vi "EZ1 MB1010 Sonar - Digital.vi"() -> ()   [LabVIEW 2013]
doc: "This example shows how to use the MaxBotix LV-MaxSonar-EZ1 Sonar Range Finder MB1010. It will display the distance from the sensor in inches.\n\nThis example works with the NI 9403 module connected to a Digital Sidecar. The Digital Sidecar should have 12V applied to the WAGO connector. The sensor is attached to the 3x8 header using a 3-pin PWM connector."
uses:
  <vilib>/Rock Robotics/SystemInterfaces/DIO/FPGA_DIOChannel.ctl
  <vilib>/Rock Robotics/SystemInterfaces/Typedef/FPGA_TypedefDigitalModule.ctl
  <vilib>/Rock Robotics/WPI/Counter/WPI_CounterDigitalInputToDigitalSource.vi
  <vilib>/Rock Robotics/WPI/Counter/WPI_CounterOpen Semi Period Mode.vi
panel:
  out "distance":dbl(slide)=125.0 scale=0.0..250.0 scale format="%3d"
  in  "Scaling factor (s/in)":dbl=0.000147
  in  "DIO Module":T1
  in  "DIO Channel":T2=enum."DIO 11"
  in  "stop":bool
  # "Set these inputs before running."
  # "This can be set while runnning."
  # "Wiring Diagram for Digital Sidecar connected to an NI 9403"
  # "PWR"
  # "SIG"
  # "(-)"
  # "14\n13\n12\n11\n10\n9\n8\n7\n6\n5\n4\n3\n2\n1"
  # "EZ1 MB1010"
  # "DIGITAL I/O"
  # "This shows wiring for a MaxBotix LV-MaxSonar-EZ1 Sonar Range Finder MB1010."
  # "GND"
  # "+5"
  # "TX"
  # "RX"
  # "AN"
  # "PW"
  # "BW"
  # "Digital Sidecar"
  # "Output information."
  # "EZ1"
  # "inches"
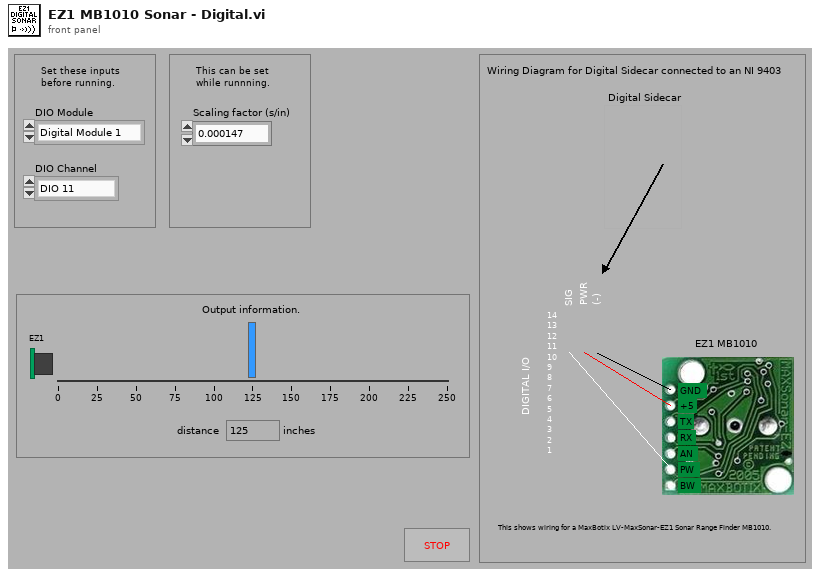
[diagram p1: front panel]
types:
  T1 = typedef "FPGA_TypedefDigitalModule.ctl" = enum16{"Digital Module 1", "Digital Module 2"}
  T2 = typedef "FPGA_DIOChannel.ctl" = enum8{"DIO 1", "DIO 2", "DIO 3", "DIO 4", "DIO 5", "DIO 6", "DIO 7", "DIO 8", "DIO 9", "DIO 10", "DIO 11", "DIO 12", "DIO 13", "DIO 14", "Invalid"}
  T3 = typedef "WPI_DigitalInputDevRef.ctl" = cluster{"DevStatus":errorcluster, "DIO Channel":T2, "Digital Module":T1}
  T4 = typedef "FPGA_CounterEncoderSourceConvertionLVSourceType.ctl" = cluster{"DevStatus":errorcluster, "AnalogTriggerMode?":bool, "DigitalMode":cluster{"Digital Module":T1, "DIO Channel":T5}, "AnalogTriggerMode":cluster{"AnalogTriggerIndex":T6, "OutputType":T7}}
  T5 = typedef "FPGA_DIODigitalSourceChannel.ctl" = enum8{"DIO 1", "DIO 2", "DIO 3", "DIO 4", "DIO 5", "DIO 6", "DIO 7", "DIO 8", "DIO 9", "DIO 10", "DIO 11", "DIO 12", "DIO 13", "DIO 14", "Disabled"}
  T6 = typedef "FPGA_AnalogTriggerIndex.ctl" = enum8{"Trig 0", "Trig 1", "Trig 2", "Trig 3", "Trig 4", "Trig 5", "Trig 6", "Trig 7", "Invalid"}
  T7 = typedef "FPGA_AnalogTriggerOutType.ctl" = enum16{"InWindow", "TriggerState", "Rising", "Falling"}
  T8 = typedef "WPI_CounterDevRef.ctl" = cluster{"DevStatus":errorcluster, "CntIndex":T9}
  T9 = typedef "FPGA_CounterCtrSystemIndex.ctl" = enum8{"Ctr 0", "Ctr 1", "Ctr 2", "Ctr 3", "Ctr 4", "Ctr 5", "Ctr 6", "Ctr 7", "Invalid"}
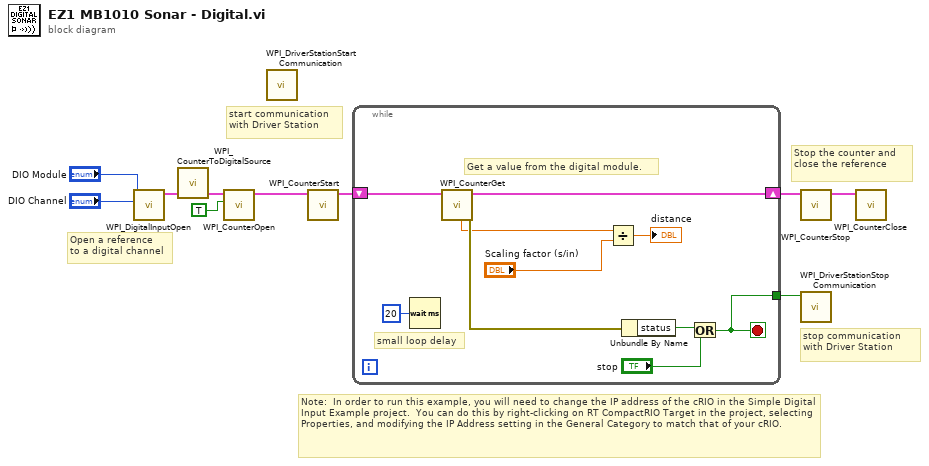
[diagram p0: block diagram]
diagram:
  # "stop communication with Driver Station"
  # "start communication with Driver Station"
  # "Note:  In order to run this example, you will need to change the IP address of the cRIO in the Simple Digital Input Example project.  You can do this by right-clicking on RT CompactRIO Target in the project, selecting Properties, and modifying the IP Address setting in the General Category to match that of your cRIO."
  # "Stop the counter and close the reference"
  # "Open a reference\nto a digital channel"
  n1 = call <vilib>:"WPI_DigitalInputOpen.vi"("DIO Channel"="DIO Channel", "Digital Module (Module 1)"="DIO Module") -> ("DigitalInputDevRef"=w5:T3)  [unwired: 1 in, 8 out]
  n2 = call-poly <vilib>:"WPI_CounterToDigitalSource.vi"("DigitalInputDevRef"=w5) -> ("Digital Source"=w7:T4)  [unwired: 6 in]
  n3 = call-poly <vilib>:"WPI_CounterOpen.vi"("High Pulse (T)"=TRUE, "Source"=w7) -> ("CounterDevRef"=w6:T8)  [unwired: 8 in, 1 out]
  n4 = call <vilib>:"WPI_DriverStationStart Communication.vi"() -> ()  [unwired: 1 in, 11 out]
  n5 = call <vilib>:"WPI_CounterStart.vi"("CounterDevRef in"=w6) -> ("CounterDevRef out"=w4:T8)  [unwired: 9 in, 1 out]
  n6 = while {
    shift-right: [w19] -> w3
    shift-left: w4 -> [w20]
    tunnel: [w16] -> w9
    stop <- w16 stop-if-true
    # "small loop delay"
    # "Get a value from the digital module."
    n7 = Wait (ms)(milliseconds to wait=u32 20) -> ()  [unwired: 1 out]
    n8 = call <vilib>:"WPI_CounterGet.vi"("CounterDevRef in"=w20) -> ("error out"=w15:errorcluster, "CounterDevRef out"=w19:T8, "Period (sec)"=w13:dbl)  [unwired: 5 in, 3 out]
    n9 = Divide(x=w13, y="Scaling factor (s/in)") -> (x/y=→"distance":dbl)
    n10 = Unbundle By Name(w15) -> ("status"=w17:bool)
    n11 = Or(x=w17, y="stop") -> (x .or. y?=w16:bool)
  }
  n12 = call <vilib>:"WPI_CounterStop.vi"("CounterDevRef in"=w3) -> ("CounterDevRef out"=w2:T8)  [unwired: 9 in, 1 out]
  n13 = call <vilib>:"WPI_DriverStationStop Communication.vi"("StopCommunication"=w9) -> ()  [unwired: 1 in, 10 out]
  n14 = call <vilib>:"WPI_CounterClose.vi"("CounterDevRef"=w2) -> ()  [unwired: 10 in, 1 out]
